vi "Write Image Format.vi"(8 "error in (no error)":errorcluster, 10 "Image Format":T1, 11 "MSOX6004 in":refnum<class "MSOX6004.lvclass">) -> (0 "error out":errorcluster, 3 "MSOX6004 out":refnum<class "MSOX6004.lvclass">)   [LabVIEW 2018, in "MSOX6004.lvlib" / "MSOX6004.lvclass"]
uses:
  MSOX6004.lvclass
  Custom Controls/Image Format.ctl
  MSOX6004.lvclass/MSOX6004.ctl
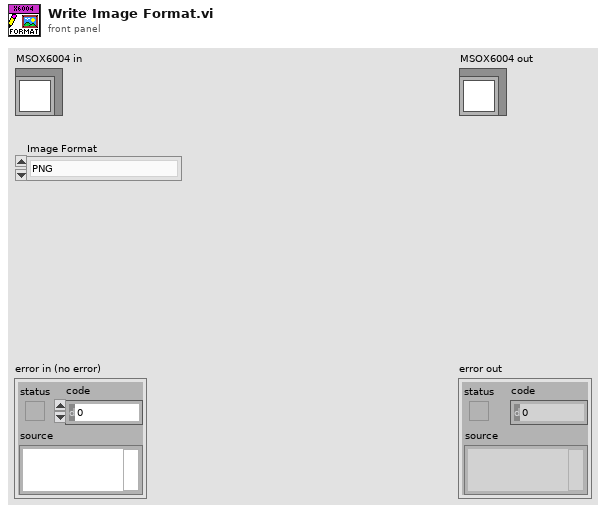
[diagram p1: front panel]
types:
  T1 = typedef "MSOX6004.lvlib/MSOX6004.lvclass/Image Format.ctl" = enum16{"PNG", "BMP"}
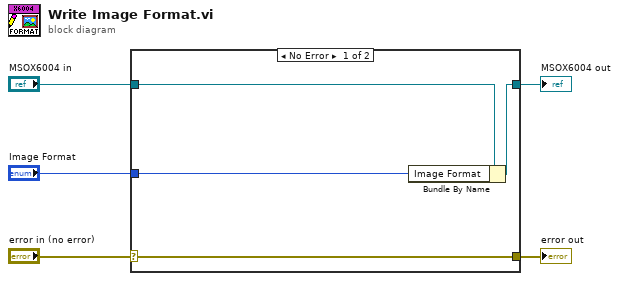
[diagram p0: block diagram]
diagram:
  n1 = case shown="No Error" "error in (no error)" {
    selector: "error in (no error)" -> [w9 w10]
    tunnel: [w9 w10] -> w4
    tunnel: [w7 w11] -> w2
    tunnel: "MSOX6004 in" -> [w8 w11]
    tunnel: "Image Format" -> [w6 _]
    frame No Error {
      n2 = Bundle By Name(cluster=w8, "Image Format"=w6) -> (w7:refnum<class "MSOX6004.lvclass">)
    }
    frame Error {
    }
  }
  "error out" <- w4
  "MSOX6004 out" <- w2
